vi "Memory Management.MoveDblBlock.Read (Double).vi"(0 "src in":dbl[](array[numeric]), 1 "src index (0)":u64, 2 "dst ptr in":u64, 3 "dst offset (0)":u64, 4 "count":i64, 5 "error in (no error)":errorcluster) -> (14 "src out":dbl[](array[numeric]), 15 "src index out":u64, 16 "dst ptr out":u64, 17 "dst offset out":u64, 18 "count out":i64, 19 "error out":errorcluster)   [LabVIEW 2016, in "VeriStand Data.lvlib"]
doc: "Calls into VeriStand's Data Services library to move a data block of length <B>size</B> from the <B>src</B> to <B>dst</B>."
uses:
  VeriStand Data.lvlib
  <vilib>/NI Veristand/Custom Device API/data/NIVeriStand_DataServices.dll
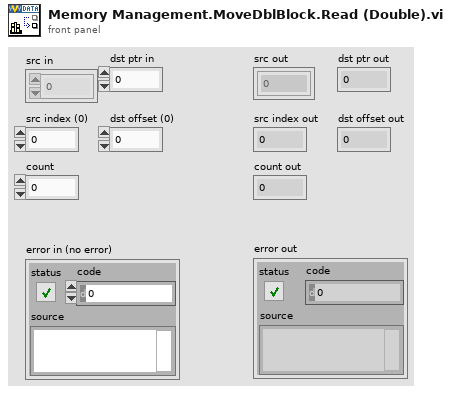
[diagram p1: front panel]
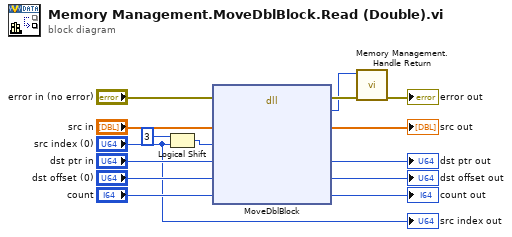
[diagram p0: block diagram]
diagram:
  n1 = Logical Shift(y=i16 3, x="src index (0)") -> (x << y=w8:u64)
  n2 = dll-call lib="C:/Program Files (x86)/National Instruments/LabVIEW 2016/vi.lib/NI Veristand/Custom Device API/data/NIVeriStand_DataServices.*" fn="MoveDblBlock"(error in="error in (no error)", "srcPtr"="src in", "srcOffset"=w8, "dstPtr"="dst ptr in", "dstOffset"="dst offset (0)", "count"="count") -> (error out=w6:errorcluster, "return type"=w4:i32, "srcPtr"=→"src out":dbl[], "dstPtr"=→"dst ptr out":u64, "dstOffset"=→"dst offset out":u64, "count"=→"count out":i64)  [unwired: 3 in, 1 out]
  n3 = call "Memory Management.Handle Return.vi"("error in (no error)"=w6, "return"=w4) -> ("error out"=→"error out":errorcluster)  [unwired: 9 in]
  "src index out" <- "src index (0)"
